vi "create_pie_legend.vi"   [LabVIEW 2024]
types:
  T1 = cluster{"Immatricule":string, "Color":u32, bool}[]
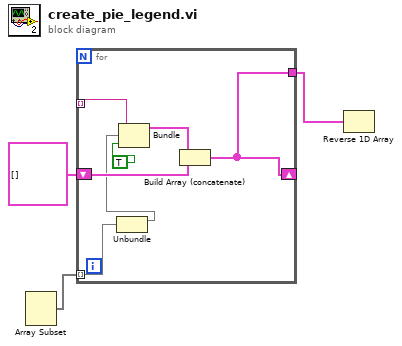
[diagram p0: block diagram]
diagram:
  n1 = Array Subset() -> (w3:void[])  [unwired: 3 in]
  n2 = for {
    tunnel: [w11] -> w4 mode=indexing
    shift-right: [w8] -> _
    shift-left: T1 [] -> [w9]
    tunnel: [w8] -> w1
    tunnel: w3 -> [w5] mode=indexing
    n3 = Unbundle(w5) -> (w6)  [unwired: 1 out]
    n4 = Bundle(w11, w6, TRUE) -> (w10:cluster{void, void, bool})  [unwired: 1 in]
    n5 = Build Array (concatenate)(w10, w9) -> (w8:T1)
  }
  n6 = Reverse 1D Array(array=w1) -> ()  [unwired: 1 out]
